vi "Keithley 2400 LDR Aug 27 2024.vi"() -> ()   [LabVIEW 2023]
uses:
  <vilib>/Analysis/1siggen.llb/Ramp Pattern by Samples.vi
  <vilib>/Analysis/baseanly.llb/Mean (DBL).vi
  <instrlib>/Keithley 24XX/Public/Data/Read (Multiple Points).vi
  <vilib>/Utility/file.llb/Write Delimited Spreadsheet (DBL).vi
  <instrlib>/Keithley 24XX/Keithley 24XX.lvlib
  <vilib>/Analysis/NI_AALBase.lvlib
panel:
  in  "type":u16(ring)=1 items=["Linear", "Logarithmic"]
  out "Lamp % vs Photocurrent":cluster{"Y":dbl[], "Y":dbl[]}[](graph)=[{"Y"=array[400 elements], "Y"=[7.624897477853664e-08, 8.58554827232183e-08, 9.090039227999114e-08, 9.412896844196439e-08, 9.633901356664865e-08, 9.788187824710803e-08, 9.898800641394701e-08, 9.981059960750826e-08, 1.0039935389727362e-07, 1.0088645225891924e-07, 1.0131995011875006e-07, 1.0178040881214656e-07, 1.0234107676865278e-07, 1.0308206128684106e-07, 1.0411798712084419e-07, 1.0556579965737001e-07, 1.0755872779100172e-07, 1.1023797554798876e-07, 1.1376307895716309e-07, 1.1821744152484826e-07]}]
  in  "file path (dialog if empty)":path=path "G:/.shortcut-targets-by-id/1Kj_JwS6Cfwfqaz0ugzl18DK49iv9Rs0M/Equipment + Data/DC2200 Measurements/HgTe SPLE Phillipe BA MpOH HgCl2/LDR.txt"
  in  "Number of Points":i32=20
  in  "Compliance  Level (0.1)":dbl=0.1
  in  "Highest Light Power":dbl=1000.0 format="%0.2f"
  in  "Lowest Light Power":dbl=1.0 format="%0.6f"
  in  "Keithley Voltage (V)":dbl=0.5
  in  "Terminal (10A 12 Pin)":u16(ring)=2 items=["10A 12 Pin"=1, "2A 4 Pin"=2]
  in  "Select LED Driver":refnum<visa-resource-name>="USB0::0x1313::0x80C8::M00982628::INSTR"
  in  "Measurement Speed (s)":dbl=5.0 format="%.2g"
  in  "Compliance Level":dbl=0.1
  in  "Keithley":refnum<visa-resource-name>="GPIB0::21::INSTR"
  # "Keithley Controls"
  # "LED Controls"
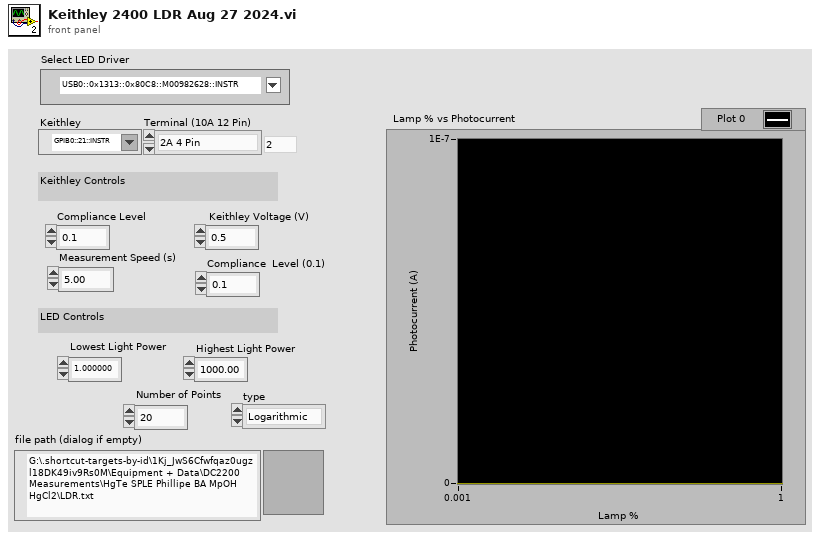
[diagram p1: front panel]
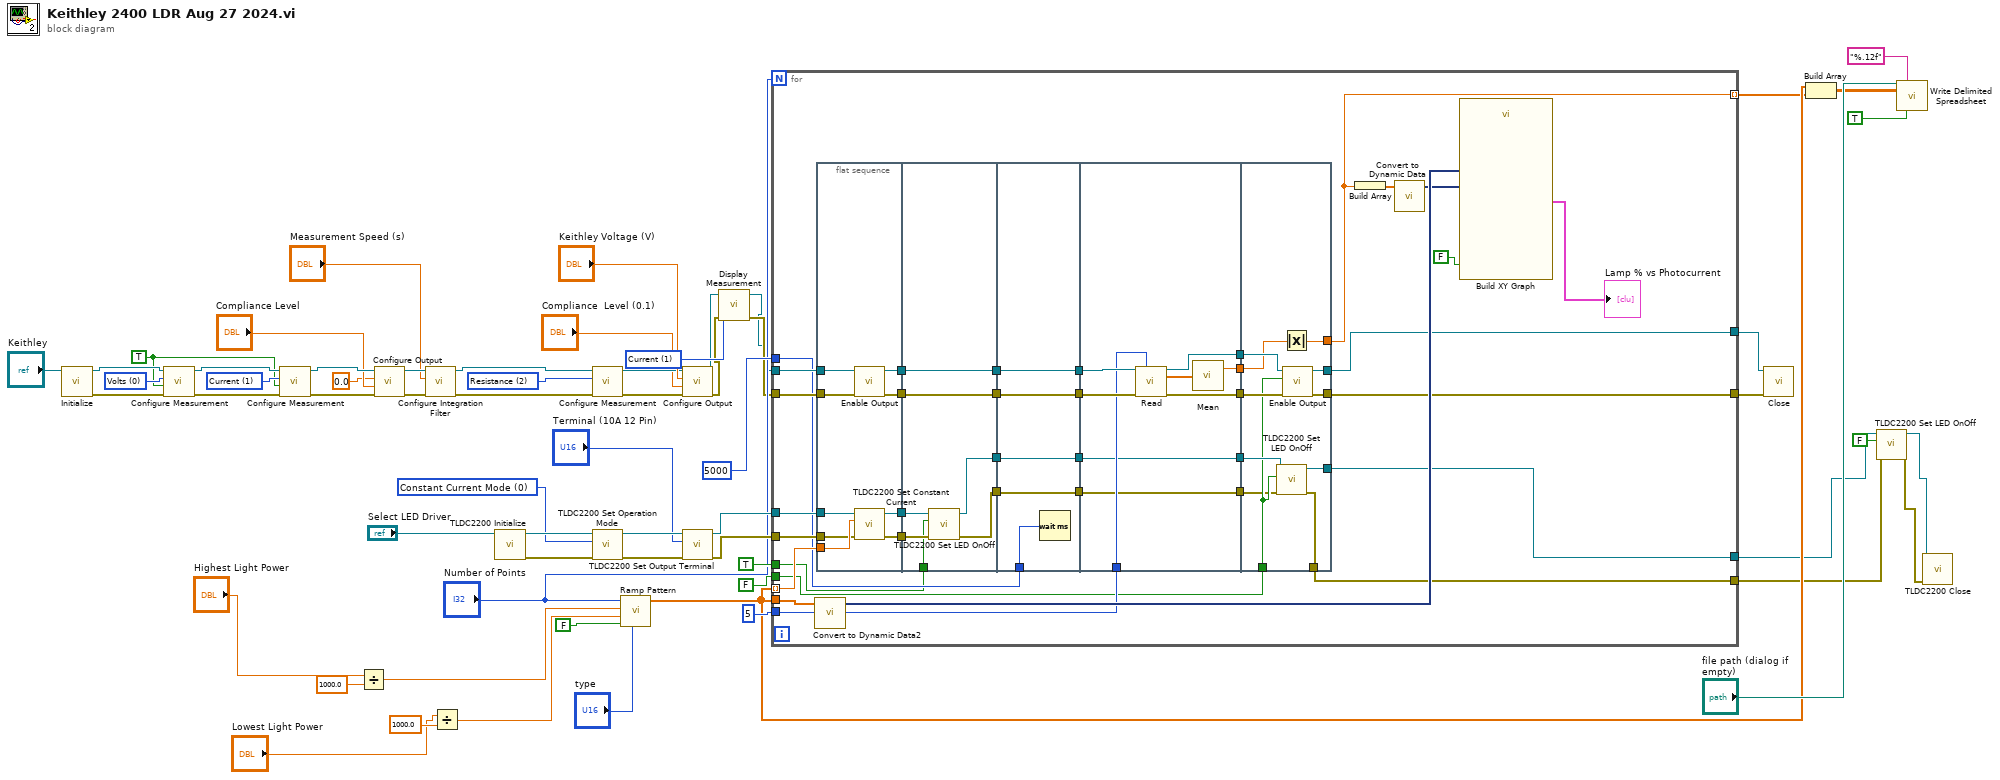
[diagram p0: block diagram]
diagram:
  w12 = u16 1 items=["Voltage", "Current", "Resistance"] ("Displayed Measurement (0: Voltage)")
  w39 = u16 2 items=["Volts", "Current", "Resistance"] ("Function (0: Volts)")
  w44 = 0 items=["Constant Current Mode", "PWM Mode", "External Modulation Mode", "Constant Brightness Mode", "Pulse Mode", "Internal Modulation Mode", "TTL Mode"] ("Operation Mode")
  w55 = TRUE
  w58 = u16 1 items=["Volts", "Current", "Resistance"] ("Function (0: Volts)")
  w59 = u16 0 items=["Volts", "Current", "Resistance"] ("Function (0: Volts)")
  n1 = call <instrlib>:"Initialize.vi"("VISA resource name"="Keithley") -> ("error out"=w57:errorcluster, "VISA resource name out"=w61:refnum<visa-resource-name>)  [unwired: 9 in]
  n2 = call <instrlib>:"Configure Measurement.vi"("error in (no error)"=w57, "Enable Auto Range (T:Enable)"=w55, "Function (0: Volts)"=w59, "VISA resource name"=w61) -> ("error out"=w56:errorcluster, "VISA resource name out"=w60:refnum<visa-resource-name>)  [unwired: 6 in]
  n3 = call <instrlib>:"Configure Measurement.vi"("error in (no error)"=w56, "Enable Auto Range (T:Enable)"=w55, "Function (0: Volts)"=w58, "VISA resource name"=w60) -> ("error out"=w53:errorcluster, "VISA resource name out"=w54:refnum<visa-resource-name>)  [unwired: 6 in]
  n4 = Divide(x="Highest Light Power", y=1000.0) -> (x/y=w4:dbl)
  n5 = call <instrlib>:"Configure Output.vi"("error in (no error)"=w53, "Compliance  Level (0.1)"="Compliance Level", "Output Level (0)"=0.0, "VISA resource name"=w54) -> ("error out"=w50:errorcluster, "VISA resource name out"=w51:refnum<visa-resource-name>)  [unwired: 6 in]
  n6 = call <instrlib>:"Configure Integration Filter.vi"("error in (no error)"=w50, "Measurement Speed (1 PLC)"="Measurement Speed (s)", "VISA resource name"=w51) -> ("error out"=w38:errorcluster, "VISA resource name out"=w40:refnum<visa-resource-name>)  [unwired: 7 in]
  n7 = Divide(x="Lowest Light Power", y=1000.0) -> (x/y=w1:dbl)
  n8 = call <instrlib>:"TLDC2200 Initialize.vi"("resource name"="Select LED Driver") -> ("error out"=w46:errorcluster, "instrument handle out"=w45:refnum<visa-resource-name>)  [unwired: 9 in]
  n9 = call <instrlib>:"Configure Measurement.vi"("error in (no error)"=w38, "Function (0: Volts)"=w39, "VISA resource name"=w40) -> ("error out"=w35:errorcluster, "VISA resource name out"=w36:refnum<visa-resource-name>)  [unwired: 7 in]
  n10 = call <instrlib>:"TLDC2200 Set Operation Mode.vi"("error in (no error)"=w46, "Operation Mode (Constant Current Mode)"=w44, "instrument handle"=w45) -> ("error out"=w43:errorcluster, "instrument handle out"=w42:refnum<visa-resource-name>)  [unwired: 7 in]
  n11 = call-poly <vilib>:"Ramp Pattern.vi"("type"="type", "exclude end?"=FALSE, "start"=w1, "end"=w4, "samples"="Number of Points") -> ("Ramp Pattern"=w19:dbl[])  [unwired: 5 in, 1 out]
  n12 = call <instrlib>:"Configure Output.vi"("error in (no error)"=w35, "Compliance  Level (0.1)"="Compliance  Level (0.1)", "Output Level (0)"="Keithley Voltage (V)", "VISA resource name"=w36) -> ("error out"=w10:errorcluster, "VISA resource name out"=w11:refnum<visa-resource-name>)  [unwired: 6 in]
  n13 = call <instrlib>:"TLDC2200 Set Output Terminal.vi"("error in (no error)"=w43, "Terminal (10A 12 Pin)"="Terminal (10A 12 Pin)", "instrument handle"=w42) -> ("error out"=w32:errorcluster, "instrument handle out"=w33:refnum<visa-resource-name>)  [unwired: 7 in]
  n14 = call <instrlib>:"Display Measurement.vi"("error in (no error)"=w10, "Displayed Measurement (0: Voltage)"=w12, "VISA resource name"=w11) -> ("error out"=w9:errorcluster, "VISA resource name out"=w8:refnum<visa-resource-name>)  [unwired: 7 in]
  n15 = for {
    N: "Number of Points" -> [_]
    tunnel: w19 -> [w97] mode=indexing
    tunnel: w33 -> [w99]
    tunnel: w32 -> [w98]
    tunnel: w19 -> [w96]
    tunnel: w8 -> [w92]
    tunnel: w9 -> [w91]
    tunnel: 5 ("Sample Count (1)") -> [w88]
    tunnel: u32 5000 ("milliseconds to wait") -> [w81]
    tunnel: TRUE ("LED On/Off (Off)") -> [w80]
    tunnel: FALSE ("Enable Output (T: Enable)") -> [w78]
    tunnel: [w75] -> w27
    tunnel: [w74] -> w26
    tunnel: [w67] -> w17
    tunnel: [w63] -> w16
    tunnel: [w72] -> w18 mode=indexing
    n16 = call "Convert to Dynamic Data2"("Array"=w96) -> ("Dynamic Data Type"=w95:dynamicdata)  [unwired: 3 in]
    n17 = flat-sequence {
      tunnel: w97 -> [w108]
      tunnel: w99 -> [w107]
      tunnel: w98 -> [w106]
      tunnel: [w105] -> w94
      tunnel: [w104] -> w93
      tunnel: w92 -> [w103]
      tunnel: w91 -> [w102]
      tunnel: [w101] -> w90
      tunnel: [w100] -> w89
      tunnel: w94 -> [w115]
      tunnel: w93 -> [w114]
      tunnel: [w113] -> w85
      tunnel: w90 -> [w113]
      tunnel: [w112] -> w83
      tunnel: w89 -> [w112]
      tunnel: w80 -> [w111]
      tunnel: [w110] -> w68
      tunnel: [w109] -> w64
      tunnel: w85 -> [w120]
      tunnel: [w120] -> w84
      tunnel: w83 -> [w119]
      tunnel: [w119] -> w82
      tunnel: w81 -> [w118]
      tunnel: [w117] -> w69
      tunnel: w68 -> [w117]
      tunnel: [w116] -> w65
      tunnel: w64 -> [w116]
      tunnel: w84 -> [w129]
      tunnel: w82 -> [w128]
      tunnel: w88 -> [w127]
      tunnel: [w125] -> w79
      tunnel: [w124] -> w77
      tunnel: [w123] -> w76
      tunnel: [w122] -> w70
      tunnel: w69 -> [w122]
      tunnel: [w121] -> w66
      tunnel: w65 -> [w121]
      tunnel: [w135] -> w72
      tunnel: w79 -> [w136]
      tunnel: w78 -> [w133]
      tunnel: w77 -> [w140]
      tunnel: w76 -> [w139]
      tunnel: [w138] -> w75
      tunnel: [w137] -> w74
      tunnel: w70 -> [w134]
      tunnel: [w132] -> w67
      tunnel: w66 -> [w131]
      tunnel: [w130] -> w63
      frame #0 {
        n18 = call <instrlib>:"Enable Output.vi"("error in (no error)"=w102, "VISA resource name"=w103) -> ("error out"=w100:errorcluster, "VISA resource name out"=w101:refnum<visa-resource-name>)  [unwired: 8 in]
        n19 = call <instrlib>:"TLDC2200 Set Constant Current.vi"("error in (no error)"=w106, "Current (0.0)"=w108, "instrument handle"=w107) -> ("error out"=w104:errorcluster, "instrument handle out"=w105:refnum<visa-resource-name>)  [unwired: 7 in]
      }
      frame #1 {
        n20 = call <instrlib>:"TLDC2200 Set LED OnOff.vi"("error in (no error)"=w114, "LED On/Off (Off)"=w111, "instrument handle"=w115) -> ("error out"=w109:errorcluster, "instrument handle out"=w110:refnum<visa-resource-name>)  [unwired: 7 in]
      }
      frame #2 {
        n21 = Wait (ms)(milliseconds to wait=w118) -> ()  [unwired: 1 out]
      }
      frame #3 {
        n22 = call-poly <instrlib>:"Read.vi"("VISA resource name"=w129, "Sample Count (1)"=w127, "error in (no error)"=w128) -> ("VISA resource name out"=w124:refnum<visa-resource-name>, "Current"=w126:sgl[], "error out"=w123:errorcluster)  [unwired: 6 in, 4 out]
        n23 = call-poly <vilib>:"Mean.vi"("X"=w126) -> ("mean"=w125:dbl)  [unwired: 1 out]
      }
      frame #4 {
        n24 = call <instrlib>:"TLDC2200 Set LED OnOff.vi"("error in (no error)"=w131, "LED On/Off (Off)"=w133, "instrument handle"=w134) -> ("error out"=w130:errorcluster, "instrument handle out"=w132:refnum<visa-resource-name>)  [unwired: 7 in]
        n25 = Absolute Value(x=w136) -> (abs(x)=w135:dbl)
        n26 = call <instrlib>:"Enable Output.vi"("error in (no error)"=w139, "Enable Output (T: Enable)"=w133, "VISA resource name"=w140) -> ("error out"=w137:errorcluster, "VISA resource name out"=w138:refnum<visa-resource-name>)  [unwired: 7 in]
      }
    }
    n27 = Build Array(w72) -> (w87:dbl[])
    n28 = call "Convert to Dynamic Data"("Array"=w87) -> ("Dynamic Data Type"=w86:dynamicdata)  [unwired: 3 in]
    n29 = call "Build XY Graph"("Reset"=FALSE, "Y Input"=w86, "X Input"=w95) -> ("XY Graph"=→"Lamp % vs Photocurrent":cluster{"Y":dbl[], "Y":dbl[]}[])  [unwired: 7 in, 1 out]
  }
  n30 = call <instrlib>:"Close.vi"("error in (no error)"=w26, "VISA resource name"=w27) -> ()  [unwired: 9 in, 1 out]
  n31 = Build Array(w19, w18) -> (w20:dbl[][])
  n32 = call <instrlib>:"TLDC2200 Set LED OnOff.vi"("error in (no error)"=w16, "LED On/Off (Off)"=FALSE, "instrument handle"=w17) -> ("error out"=w15:errorcluster, "instrument handle out"=w14:refnum<visa-resource-name>)  [unwired: 7 in]
  n33 = call-poly <vilib>:"Write Delimited Spreadsheet.vi"("file path (dialog if empty)"="file path (dialog if empty)", "format (%.3f)"="%.12f", "2D data"=w20, "transpose? (no:F)"=TRUE) -> ()  [unwired: 10 in, 2 out]
  n34 = call <instrlib>:"TLDC2200 Close.vi"("error in (no error)"=w15, "instrument handle"=w14) -> ()  [unwired: 9 in, 1 out]
